vi "Set Object Pointer.vi"(10 "Object Pointer":i64, 11 "Event in":refnum<class "Event.lvclass">) -> (3 "Event out":refnum<class "Event.lvclass">)   [LabVIEW 2013, in "MDSplus.lvlib" / "Event.lvclass"]
uses:
  <vilib>/MDSplus/Classes/Event_Class/Event.lvclass
  <vilib>/MDSplus/Classes/Event_Class/Event.lvclass/Event.ctl
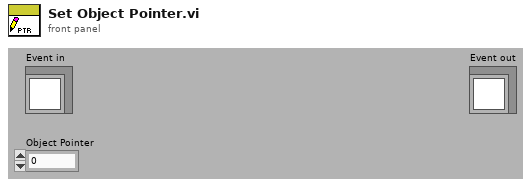
[diagram p1: front panel]
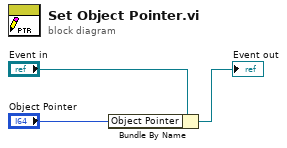
[diagram p0: block diagram]
diagram:
  n1 = Bundle By Name(cluster="Event in", "Object Pointer"="Object Pointer") -> (→"Event out":refnum<class "Event.lvclass">)
